vi "dispense test.vi"() -> ()   [LabVIEW 2018]
uses:
  Classes/Controller/Controller.lvclass
  Classes/Controller/Dispenser/Dispenser.lvclass
  C:/Users/HEP/Documents/GitHub/UCSB-Gantry-HEP-2018/Classes/Controller/Controller.lvclass
panel:
  out "Dispense on":bool
  out "error out":errorcluster
  in  "error in (no error)":errorcluster
  in  "Pressure":i16=20
  in  "Dispense":bool
  in  "stop":bool
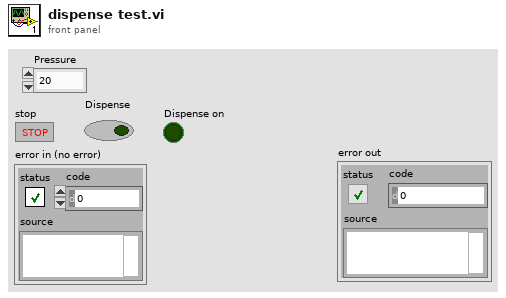
[diagram p1: front panel]
types:
  T1 = typedef "Controller.lvclass/Controllers.ctl" = cluster{"I-O.lvclass":refnum<class "I-O.lvclass">, "Gantry":refnum<k24>, "Dispenser":refnum<visa-resource-name>}
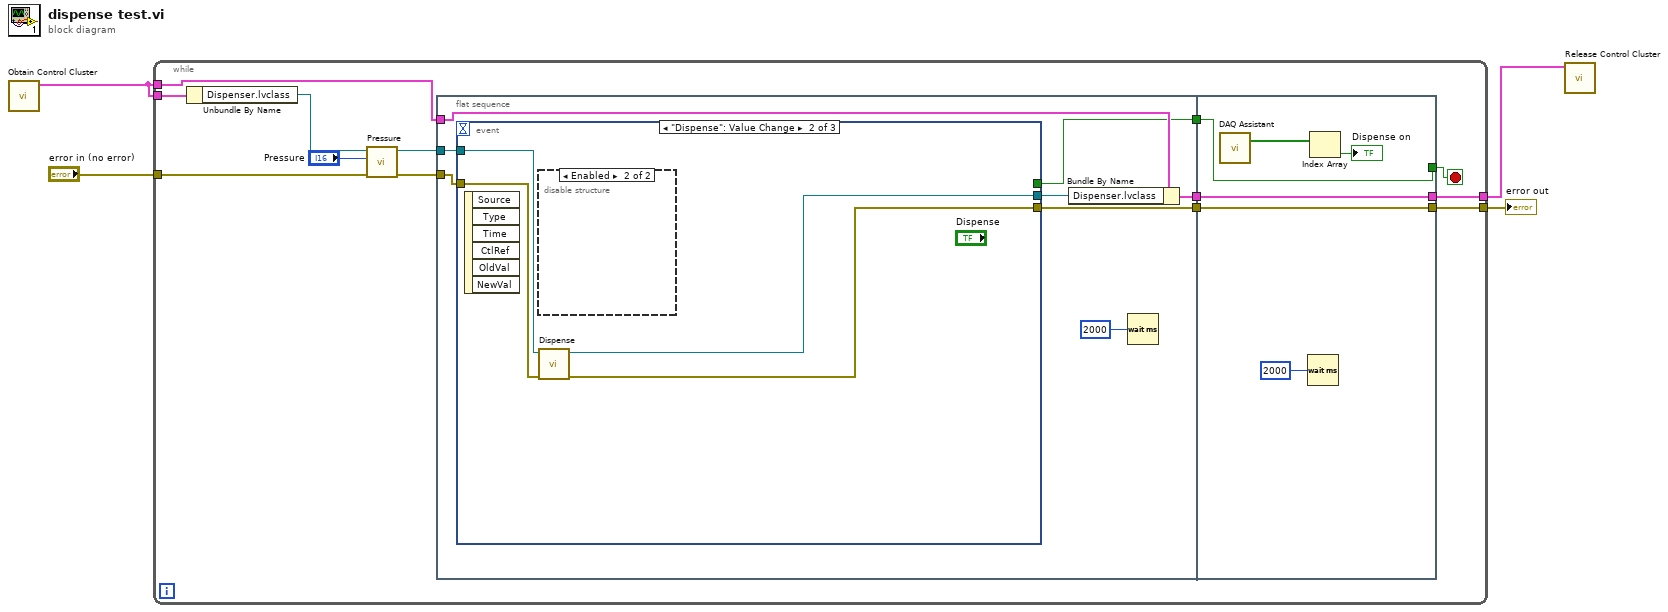
[diagram p0: block diagram]
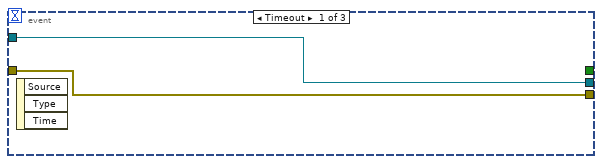
[diagram p2: hidden frame]
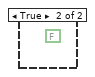
[diagram p4: hidden frame]
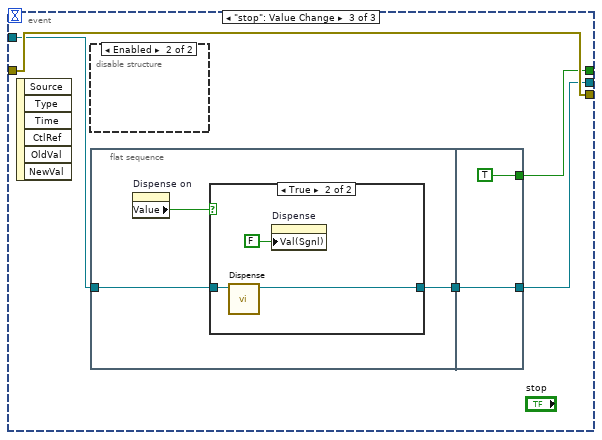
[diagram p5: hidden frame]
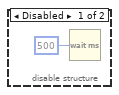
[diagram p6: hidden frame]
diagram:
  n1 = call "Obtain Control Cluster.vi"() -> ("Control Out"=w3:T1)  [unwired: 11 in]
  n2 = while {
    tunnel: w3 -> [w17]
    tunnel: "error in (no error)" -> [w14]
    tunnel: w3 -> [w12]
    tunnel: [w11] -> w2
    tunnel: [w9] -> w1
    stop <- w8 stop-if-true
    n3 = Unbundle By Name(w17) -> ("Dispenser.lvclass"=w16:refnum<class "Dispenser.lvclass">)
    n4 = call "Pressure.vi"("error in (no error)"=w14, "Pressure"="Pressure", "VISA resource name"=w16) -> ("error out"=w10:errorcluster, "VISA resource name out"=w13:refnum<visa-resource-name>)  [unwired: 7 in]
    n5 = flat-sequence {
      tunnel: w13 -> [w25]
      tunnel: w12 -> [w23]
      tunnel: w10 -> [w21]
      tunnel: [w22] -> w7
      tunnel: [w20] -> w6
      tunnel: [w19] -> w5
      tunnel: [w50] -> w8
      tunnel: [w51] -> w9
      tunnel: [w52] -> w11
      tunnel: w7 -> [w52]
      tunnel: w6 -> [w51]
      tunnel: w5 -> [w50]
      frame #0 {
        n6 = event shown="[1] \"Dispense\": Value Change" {
          selector: _ -> [_ _ _]
          dyn-events: _ -> [_ _ _]
          timeout: _ -> [_ _ _]
          tunnel: w25 -> [w27 w31 w36]
          tunnel: [w27 w30 w35] -> w24
          tunnel: w21 -> [w26 w29 w37]
          tunnel: [w26 w28 w37] -> w20
          tunnel: [_ _ w33] -> w19
          event Timeout {
            n7 = event-data() -> ()  [unwired: 1 in, 3 out]
          }
          event "Dispense": Value Change {
            n8 = event-data() -> ()  [unwired: 1 in, 6 out]
            n9 = disable-structure shown="Enabled" {
              frame Disabled {
                n10 = case shown="False" {
                  selector: _ -> [_ _]
                  frame False {
                  }
                  frame True {
                    w32 = FALSE
                  }
                }
              }
              frame Enabled {
              }
            }
            n11 = call "Dispense.vi"("error in (no error)"=w29, "Dispenser In"=w31) -> ("error out"=w28:errorcluster, "Dispenser Out"=w30:refnum<visa-resource-name>)  [unwired: 8 in]
          }
          event "stop": Value Change {
            n12 = event-data() -> ()  [unwired: 1 in, 6 out]
            n13 = disable-structure shown="Enabled" {
              frame Disabled {
                n14 = Wait (ms)(milliseconds to wait=u32 500) -> ()  [unwired: 1 out]
              }
              frame Enabled {
              }
            }
            n15 = flat-sequence {
              tunnel: w36 -> [w41]
              tunnel: [w40] -> w34
              tunnel: [w46] -> w35
              tunnel: w34 -> [w46]
              tunnel: [TRUE] -> w33
              frame #0 {
                n16 = property on="Dispense on" class="Bool (strict)"() -> ("Value"=w39:bool)  [unwired: 2 in, 2 out]
                n17 = case shown="True" w39 {
                  tunnel: w41 -> [_ w44]
                  tunnel: [_ w43] -> w40
                  frame False {
                  }
                  frame True {
                    n18 = call "Dispense.vi"("Dispenser In"=w44) -> ("Dispenser Out"=w43:refnum<visa-resource-name>)  [unwired: 9 in, 1 out]
                    n19 = property on="Dispense" class="Bool (strict)"("Val(Sgnl)"=FALSE) -> ()  [unwired: 2 in, 2 out]
                  }
                }
              }
              frame #1 {
              }
            }
          }
        }
        n20 = Bundle By Name(cluster=w23, "Dispenser.lvclass"=w24) -> (w22:T1)
        n21 = Wait (ms)(milliseconds to wait=u32 2000) -> ()  [unwired: 1 out]
      }
      frame #1 {
        n22 = call "DAQ Assistant"() -> ("data"=w49:bool[])  [unwired: 17 in, 2 out]
        n23 = Wait (ms)(milliseconds to wait=u32 2000) -> ()  [unwired: 1 out]
        n24 = Index Array(array=w49) -> (element=→"Dispense on":bool)  [unwired: 1 in]
      }
    }
  }
  "error out" <- w1
  n25 = call "Release Control Cluster.vi"("output cluster"=w2) -> ()  [unwired: 11 in]
